vi "写测量tdms.vi"(8 "错误输入（无错误）":errorcluster, 10 "消息":T1, 11 "引用句柄输入":refnum<k34>) -> (0 "错误输出":errorcluster, 3 "tdms文件输出":refnum<k34>)   [LabVIEW 2012]
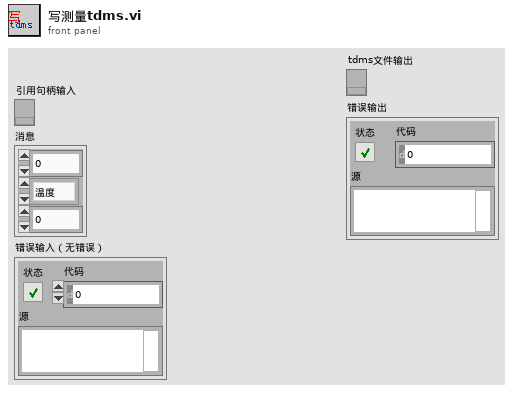
[diagram p1: front panel]
types:
  T1 = cluster{i32, enum16{"温度", "亮度", "电量", "连接质量"}, sgl}
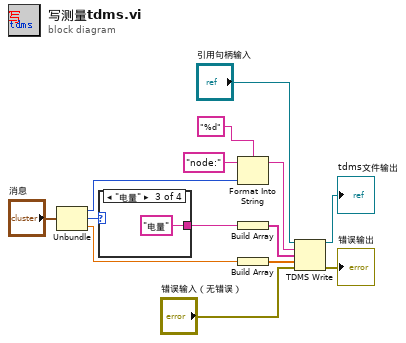
[diagram p0: block diagram]
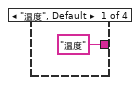
[diagram p2: hidden frame]
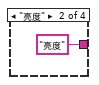
[diagram p3: hidden frame]
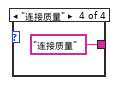
[diagram p4: hidden frame]
diagram:
  n1 = Unbundle("消息") -> (w10:i32, w7:enum16{"温度", "亮度", "电量", "连接质量"}, w4:sgl)
  n2 = case shown="\"电量\"" w7 {
    tunnel: ["温度" "亮度" "电量" "连接质量"] -> w6
    frame "温度", Default {
    }
    frame "亮度" {
    }
    frame "电量" {
    }
    frame "连接质量" {
    }
  }
  n3 = Format Into String(format string="%d" ("格式字符串"), initial string="node:", w10) -> (resulting string=w8:string)  [unwired: 1 in, 1 out]
  n4 = Build Array(w6) -> (w5:string[])
  n5 = Build Array(w4) -> (w3:sgl[])
  n6 = TDMS Write(0:"引用句柄输入", 5:w8, 7:w5, 9:w3, 11:"错误输入（无错误）") -> (4:→"tdms文件输出":refnum<k34>, 15:→"错误输出":errorcluster)  [unwired: 1 in, 2 out]
